vi "Get_RD_Files.vi"(9 "Sort RD Files? (T)":bool=TRUE, 11 "Raw Data File Folder":path) -> (3 "Array of only RD Files":path[](array[path]))   [LabVIEW 2011]
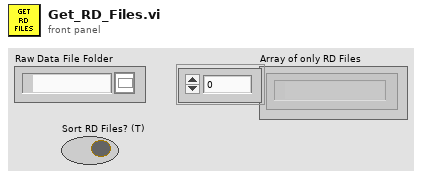
[diagram p1: front panel]
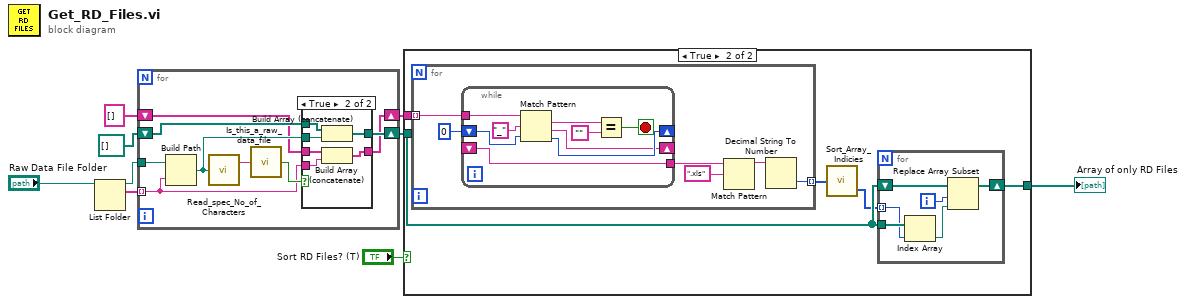
[diagram p0: block diagram]
diagram:
  n1 = List Folder(path="Raw Data File Folder") -> (path out=w3:path, filenames=w4:string[])  [unwired: 3 in, 2 out]
  n2 = for {
    tunnel: w3 -> [w17]
    tunnel: w4 -> [w12] mode=indexing
    shift-right: [w15] -> w8
    shift-left: path[] [] -> [w14]
    shift-right: [w11] -> w7
    shift-left: string[] [] -> [w10]
    n3 = Build Path(base path=w17, name or relative path=w12) -> (appended path=w16:path)
    n4 = call "Read_spec_No_of_Characters.vi"("Filename"=w16) -> ("character string"=w18:string)  [unwired: 1 out]
    n5 = call "Is_this_a_raw_data_file.vi"("character string"=w18) -> ("Raw Dat File?"=w13:bool)  [unwired: 2 out]
    n6 = case shown="True" w13 {
      tunnel: w16 -> [_ w26]
      tunnel: [w20 w24] -> w15
      tunnel: w14 -> [w20 w25]
      tunnel: w12 -> [_ w23]
      tunnel: [w19 w22] -> w11
      tunnel: w10 -> [w19 w21]
      frame False {
      }
      frame True {
        n7 = Build Array (concatenate)(w25, w26) -> (w24:path[])
        n8 = Build Array (concatenate)(w21, w23) -> (w22:string[])
      }
    }
  }
  n9 = case shown="True" "Sort RD Files? (T)" {
    tunnel: [w27 w32] -> w9
    tunnel: w8 -> [w27 w31]
    tunnel: w7 -> [_ w28]
    frame False {
    }
    frame True {
      n10 = for {
        tunnel: w28 -> [w44] mode=indexing
        tunnel: [w39] -> w29 mode=indexing
        n11 = while {
          tunnel: w44 -> [w53]
          shift-right: [w47] -> _
          shift-left: 0 ("offset past match") -> [w51]
          shift-right: [w45] -> _
          shift-left: _ -> [w48]
          tunnel: [w48] -> w41
          stop <- w49 stop-if-true
          n12 = Match Pattern(string=w53, regular expression="_", offset (0)=w51) -> (match substring=w46:string, after substring=w45:string, offset past match=w47:i32)  [unwired: 1 out]
          n13 = Equal?(x=w46, y="") -> (x = y?=w49:bool)
        }
        n14 = Match Pattern(string=w41, regular expression=".xls") -> (before substring=w40:string)  [unwired: 1 in, 3 out]
        n15 = Decimal String To Number(string=w40) -> (number=w39:i32)  [unwired: 2 in, 1 out]
      }
      n16 = call "Sort_Array_Indicies.vi"("unsorted array"=w29) -> ("Sort Index"=w30:i32[])  [unwired: 1 out]
      n17 = for {
        tunnel: w30 -> [w35] mode=indexing
        tunnel: w31 -> [w36]
        shift-right: [w34] -> w32
        shift-left: w31 -> [w38]
        i -> [w37]
        n18 = Index Array(array=w36, index=w35) -> (element=w33:path)
        n19 = Replace Array Subset(array=w38, new element=w33, index=w37) -> (w34:path[])
      }
    }
  }
  "Array of only RD Files" <- w9
